vi "ClockWatcher.vi"() -> ()   [LabVIEW 2020]
uses:
  <userlib>/caLab/Private/Get_PV-1D.vi
panel:
  out "PC Current Time":timestamp[](array[timestamp])
  in  "PC Name":string[](array[string])=["DAFFY"]
  in  "Stop":bool
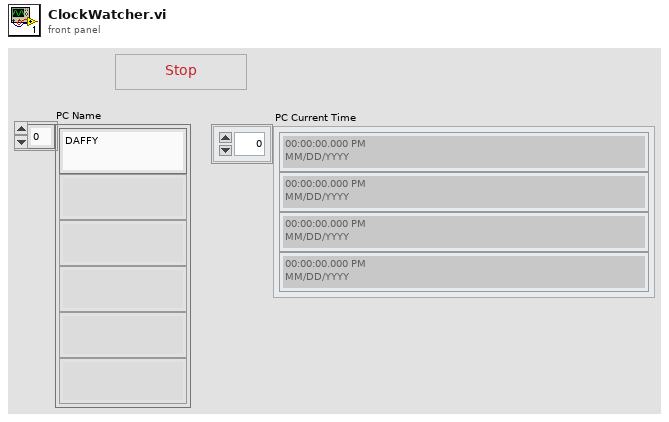
[diagram p1: front panel]
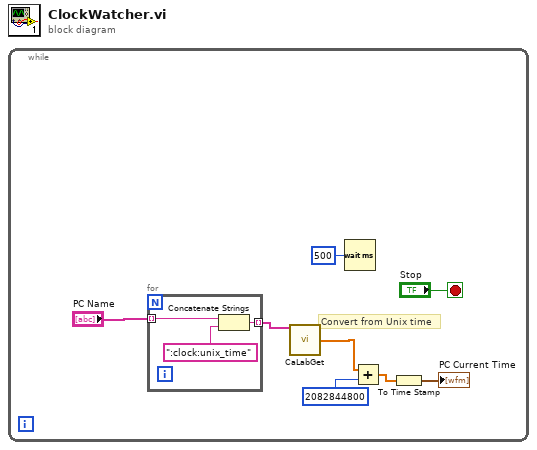
[diagram p0: block diagram]
diagram:
  n1 = while {
    stop <- "Stop" stop-if-true
    # "Convert from Unix time"
    n2 = for {
      tunnel: "PC Name" -> [w10] mode=indexing
      tunnel: [w9] -> w5 mode=indexing
      n3 = Concatenate Strings(w10, ":clock:unix_time") -> (w9:string)
    }
    n4 = call-poly <userlib>:"CaLabGet.vi"("PV Names"=w5) -> ("1rst Value (number)"=w1:dbl[])  [unwired: 8 in, 6 out]
    n5 = Wait (ms)(milliseconds to wait=u32 500) -> ()  [unwired: 1 out]
    n6 = Add(x=w1, y=2082844800) -> (x+y=w3:dbl[])
    n7 = To Time Stamp(1:w3) -> (0:→"PC Current Time":timestamp[])
  }
